vi "DCMCT_Speed_Digital_Scopes.vi"(1 "Speed (rad/s)":dbl, 2 "Current (A)":dbl) -> (0 "Digital Scopes":T1)   [LabVIEW 2010]
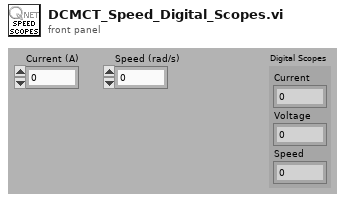
[diagram p1: front panel]
types:
  T1 = cluster{"Current":dbl, "Voltage":dbl, "Speed":dbl}
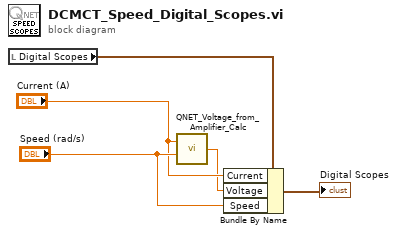
[diagram p0: block diagram]
diagram:
  n1 = local read "Digital Scopes"() -> (w1:T1)
  n2 = call "QNET_Voltage_from_Amplifier_Calc.vi"("Speed (rad/s)"="Speed (rad/s)", "Im (A)"="Current (A)") -> ("Vm (V)"=w3:dbl)
  n3 = Bundle By Name(cluster=w1, "Current"="Current (A)", "Voltage"=w3, "Speed"="Speed (rad/s)") -> (→"Digital Scopes":T1)
